vi "Get Element Index.vi"(0 "Element":string, 2 "List":string[](array[string])) -> (7 "result":i32, 9 "found?":bool)   [LabVIEW 2013, in "Helpers.lvlib"]
uses:
  Helpers.lvlib
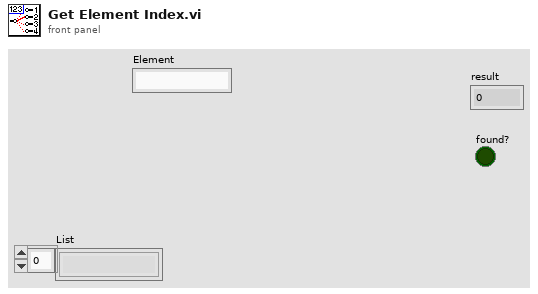
[diagram p1: front panel]
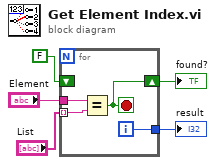
[diagram p0: block diagram]
diagram:
  n1 = for {
    tunnel: "Element" -> [w9]
    shift-right: [w8] -> w3
    shift-left: FALSE -> [_]
    tunnel: [w7] -> w2
    tunnel: "List" -> [w6] mode=indexing
    i -> [w7]
    stop <- w8 stop-if-true
    n2 = Equal?(x=w9, y=w6) -> (x = y?=w8:bool)
  }
  "found?" <- w3
  "result" <- w2
